vi "RobotDLLError(SubVI).vi"(0 "ArmID":i32, 5 "KillRobotControlProcess":bool) -> (2 "ROBOT_COMMAND_BEYONG_JOINT_RANGE":bool, 3 "ROBOT_KINEMATICS_NO_SOLUTION":bool, 4 "ROBOT_HARDWARE_NOT_PRESENT":bool, 6 "ROBOT_HARDWARE_NOT_FOUND_ALL_DRIVES":bool, 8 "ROBOT_HARDWARE_SENSOR_FAULT":bool, 10 "ROBOT_NOT_RUNNING":bool, 12 "RobotStatusArray":bool[](array[boolean]), 13 "ROBOT_COMMAND_TOO_LARGE":bool, 14 "ROBOT_KINEMATICS_INSERTION_LENGTH_TOO_SMALL":bool, 15 "ROBOT_COMMUNICATION_ERROR":bool)   [LabVIEW 2016]
uses:
  EyeRobotDLL.dll
panel:
  out "Numeric 4":i64 format="%x"
  out "Robot Status":dbl
  # "ROBOT_HARDWARE_NOT_PRESENT"
  # "ROBOT_HARDWARE_NOT_FOUND_ALL_DRIVES"
  # "ROBOT_HARDWARE_SENSOR_FAULT"
  # "ROBOT_NOT_RUNNING"
  # "ROBOT_COMMUNICATION_ERROR"
  # "ROBOT_KINEMATICS_NO_SOLUTION"
  # "ROBOT_KINEMATICS_INSERTION_LENGTH_TOO_SMALL"
  # "ROBOT_COMMAND_BEYOND_JOINT_RANGE"
  # "ROBOT_COMMAND_TOO_LARGE"
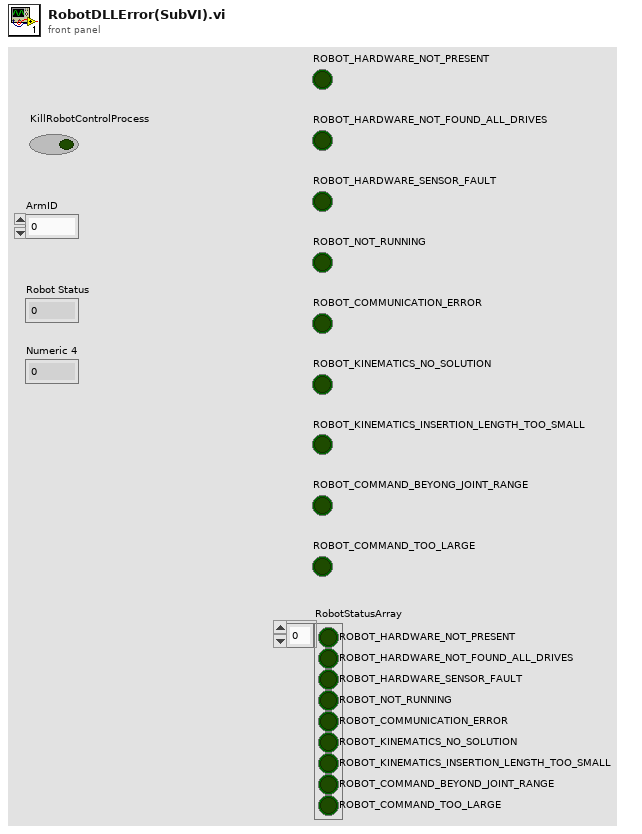
[diagram p1: front panel]
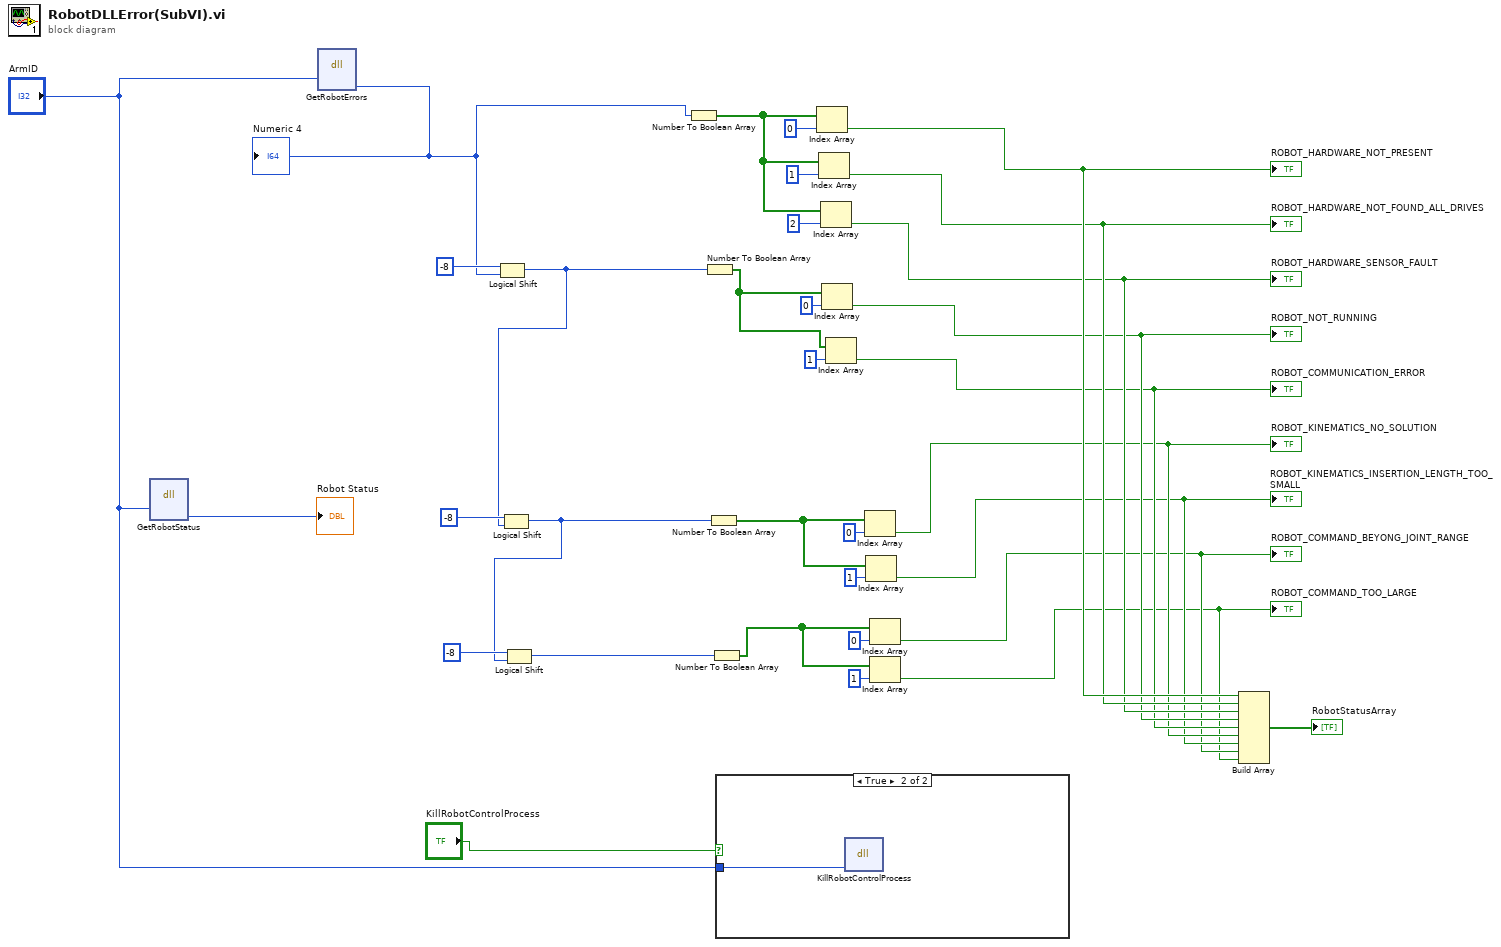
[diagram p0: block diagram]
diagram:
  n1 = dll-call lib="D:/IRISSoft LV2016 beta/Host Demo/Functions/EyeRobotDLL.dll" fn="GetRobotStatus"("id"="ArmID") -> ("status"=→"Robot Status":i32)  [unwired: 6 in, 2 out]
  n2 = dll-call lib="D:/IRISSoft LV2016 beta/Host Demo/Functions/EyeRobotDLL.dll" fn="GetRobotErrors"("id"="ArmID") -> ("errors"=w13:i32)  [unwired: 6 in, 2 out]
  "Numeric 4" <- w13
  n3 = Logical Shift(y=i16 -8, x=w13) -> (x << y=w23:i32)
  n4 = Logical Shift(y=i16 -8, x=w23) -> (x << y=w17:i32)
  n5 = Logical Shift(y=i16 -8, x=w17) -> (x << y=w18:i32)
  n6 = Number To Boolean Array(number=w13) -> (Boolean array=w28:bool[])
  n7 = Number To Boolean Array(number=w23) -> (Boolean array=w25:bool[])
  n8 = Number To Boolean Array(number=w17) -> (Boolean array=w20:bool[])
  n9 = Number To Boolean Array(number=w18) -> (Boolean array=w16:bool[])
  n10 = case shown="True" "KillRobotControlProcess" {
    tunnel: "ArmID" -> [_ w34]
    frame False {
    }
    frame True {
      n11 = dll-call lib="D:/IRISSoft LV2016 beta/Host Demo/Functions/EyeRobotDLL.dll" fn="KillRobotControlProcess"("id"=w34) -> ()  [unwired: 5 in, 2 out]
    }
  }
  n12 = Index Array(array=w28, index=0) -> (element=w10:bool)
  "ROBOT_HARDWARE_NOT_PRESENT" <- w10
  n13 = Index Array(array=w28, index=1) -> (element=w9:bool)
  "ROBOT_HARDWARE_NOT_FOUND_ALL_DRIVES" <- w9
  n14 = Index Array(array=w28, index=2) -> (element=w8:bool)
  "ROBOT_HARDWARE_SENSOR_FAULT" <- w8
  n15 = Index Array(array=w25, index=0) -> (element=w7:bool)
  "ROBOT_NOT_RUNNING" <- w7
  n16 = Index Array(array=w25, index=1) -> (element=w6:bool)
  "ROBOT_COMMUNICATION_ERROR" <- w6
  n17 = Index Array(array=w20, index=0) -> (element=w5:bool)
  "ROBOT_KINEMATICS_NO_SOLUTION" <- w5
  n18 = Index Array(array=w20, index=1) -> (element=w4:bool)
  "ROBOT_KINEMATICS_INSERTION_LENGTH_TOO_SMALL" <- w4
  n19 = Index Array(array=w16, index=0) -> (element=w3:bool)
  "ROBOT_COMMAND_BEYONG_JOINT_RANGE" <- w3
  n20 = Index Array(array=w16, index=1) -> (element=w2:bool)
  "ROBOT_COMMAND_TOO_LARGE" <- w2
  n21 = Build Array(w10, w9, w8, w7, w6, w5, w4, w3, w2) -> (→"RobotStatusArray":bool[])
